vi "Valore da riga acq.vi"(10 "Filtro":bool[](array[boolean]), 11 "RIGA":string[](array[string])) -> (3 "MISURE NM":T1)   [LabVIEW 2019]
uses:
  TypeDef/MISURE NM.ctl
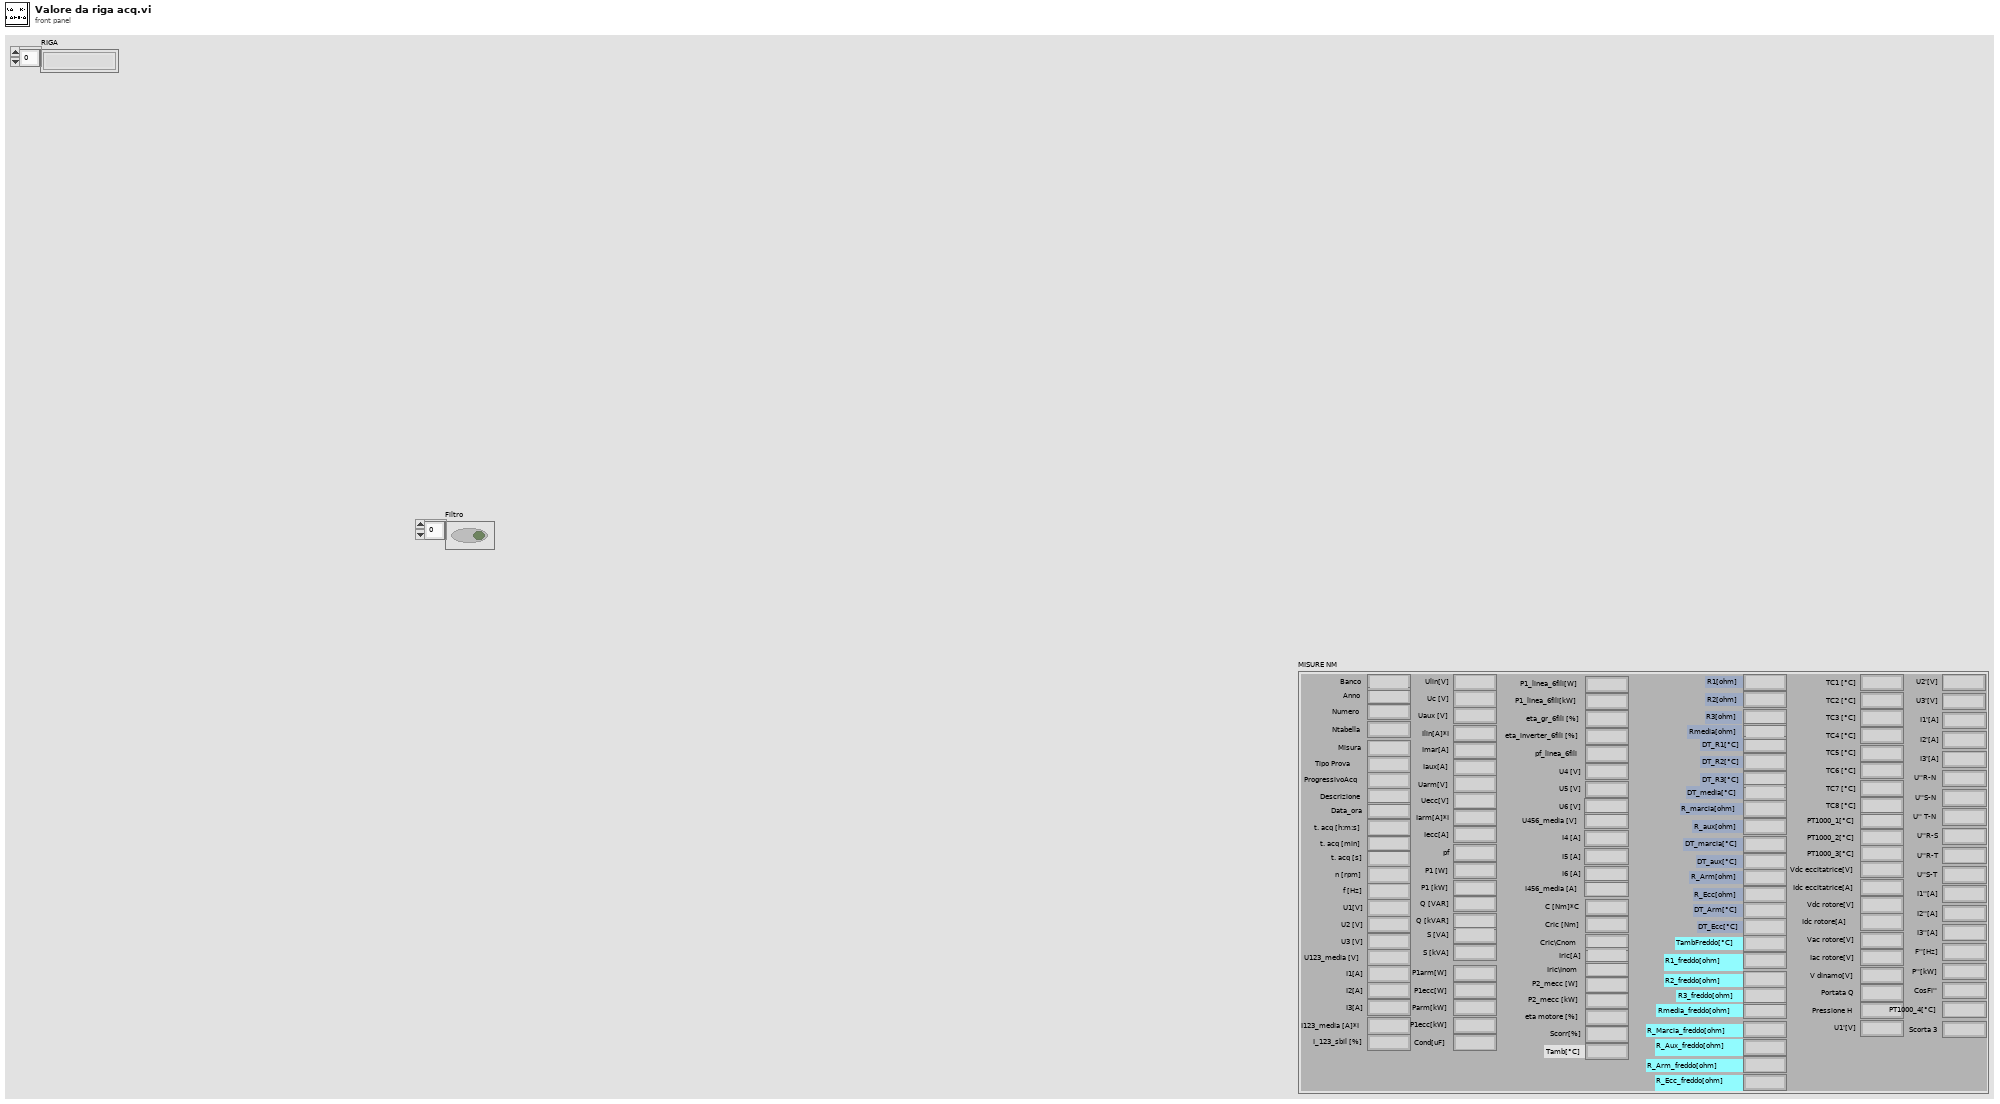
[diagram p1: front panel]
types:
  T1 = typedef "MISURE NM.ctl" = cluster{"Banco":string, "Anno":string, "Numero":string, "Ntabella":string, "Misura":string, "Tipo Prova":string, "ProgressivoAcq":string, "Descrizione":string, "Data_ora":string, "t. acq [h:m:s]":string, "t. acq [min]":string, "t. acq [s]":string, "n [rpm]":string, "f [Hz]":string, "U1[V]":string, "U2 [V]":string, "U3 [V]":string, "U123_media [V]":string, "I1[A]":string, "I2[A]":string, "I3[A]":string, "I123_media [A]*I":string, "I_123_sbil [%]":string, "Ulin[V]":string, "Uc [V]":string, "Uaux [V]":string, "Ilin[A]*I":string, "Imar[A]":string, "Iaux[A]":string, "Uarm[V]":string, "Uecc[V]":string, "Iarm[A]*I":string, "Iecc[A]":string, "pf":string, "P1 [W]":string, "P1 [kW]":string, "Q [VAR]":string, "Q [kVAR]":string, "S [VA]":string, "S [kVA]":string, "P1arm[W]":string, "P1ecc[W]":string, "Parm[kW]":string, "P1ecc[kW]":string, "Cond[uF]":string, "P1_linea_6fili[W]":string, "P1_linea_6fili[kW]":string, "eta_gr_6fili [%]":string, "eta_inverter_6fili [%]":string, "pf_linea_6fili":string, "U4 [V]":string, "U5 [V]":string, "U6 [V]":string, "U456_media [V]":string, "I4 [A]":string, "I5 [A]":string, "I6 [A]":string, "I456_media [A]":string, "C [Nm]*C":string, "Cric [Nm]":string, "Cric\\Cnom":string, "Iric[A]":string, "Iric\\Inom":string, "P2_mecc [W]":string, "P2_mecc [kW]":string, "eta motore [%]":string, "Scorr[%]":string, "Tamb[°C]":string, "R1[ohm]":string, "R2[ohm]":string, "R3[ohm]":string, "Rmedia[ohm]":string, "DT_R1[°C]":string, "DT_R2[°C]":string, "DT_R3[°C]":string, "DT_media[°C]":string, "R_marcia[ohm]":string, "R_aux[ohm]":string, "DT_marcia[°C]":string, "DT_aux[°C]":string, "R_Arm[ohm]":string, "R_Ecc[ohm]":string, "DT_Arm[°C]":string, "DT_Ecc[°C]":string, "TambFreddo[°C]":string, "R1_freddo[ohm]":string, "R2_freddo[ohm]":string, "R3_freddo[ohm]":string, "Rmedia_freddo[ohm]":string, "R_Marcia_freddo[ohm]":string, "R_Aux_freddo[ohm]":string, "R_Arm_freddo[ohm]":string, "R_Ecc_freddo[ohm]":string, "TC1 [°C]":string, "TC2 [°C]":string, "TC3 [°C]":string, "TC4 [°C]":string, "TC5 [°C]":string, "TC6 [°C]":string, "TC7 [°C]":string, "TC8 [°C]":string, "PT1000_1[°C]":string, "PT1000_2[°C]":string, "PT1000_3[°C]":string, "Vdc eccitatrice[V]":string, "Idc eccitatrice[A]":string, "Vdc rotore[V]":string, "Idc rotore[A]":string, "Vac rotore[V]":string, "Iac rotore[V]":string, "V dinamo[V]":string, "Portata Q":string, "Pressione H":string, "U1'[V]":string, "U2'[V]":string, "U3'[V]":string, "I1'[A]":string, "I2'[A]":string, "I3'[A]":string, "U''R-N":string, "U''S-N":string, "U'' T-N":string, "U''R-S":string, "U''R-T":string, "U''S-T":string, "I1''[A]":string, "I2''[A]":string, "I3''[A]":string, "F''[Hz]":string, "P''[kW]":string, "CosFi''":string, "PT1000_4[°C]":string, "Scorta 3":string}
  T2 = cluster{"[0]":string, "[1]":string, "[2]":string, "[3]":string, "[4]":string, "[5]":string, "[6]":string, "[7]":string, "[8]":string, "[9]":string, "[10]":string, "[11]":string, "[12]":string, "[13]":string, "[14]":string, "[15]":string, "[16]":string, "[17]":string, "[18]":string, "[19]":string, "[20]":string, "[21]":string, "[22]":string, "[23]":string, "[24]":string, "[25]":string, "[26]":string, "[27]":string, "[28]":string, "[29]":string, "[30]":string, "[31]":string, "[32]":string, "[33]":string, "[34]":string, "[35]":string, "[36]":string, "[37]":string, "[38]":string, "[39]":string, "[40]":string, "[41]":string, "[42]":string, "[43]":string, "[44]":string, "[45]":string, "[46]":string, "[47]":string, "[48]":string, "[49]":string, "[50]":string, "[51]":string, "[52]":string, "[53]":string, "[54]":string, "[55]":string, "[56]":string, "[57]":string, "[58]":string, "[59]":string, "[60]":string, "[61]":string, "[62]":string, "[63]":string, "[64]":string, "[65]":string, "[66]":string, "[67]":string, "[68]":string, "[69]":string, "[70]":string, "[71]":string, "[72]":string, "[73]":string, "[74]":string, "[75]":string, "[76]":string, "[77]":string, "[78]":string, "[79]":string, "[80]":string, "[81]":string, "[82]":string, "[83]":string, "[84]":string, "[85]":string, "[86]":string, "[87]":string, "[88]":string, "[89]":string, "[90]":string, "[91]":string, "[92]":string, "[93]":string, "[94]":string, "[95]":string, "[96]":string, "[97]":string, "[98]":string, "[99]":string, "[100]":string, "[101]":string, "[102]":string, "[103]":string, "[104]":string, "[105]":string, "[106]":string, "[107]":string, "[108]":string, "[109]":string, "[110]":string, "[111]":string, "[112]":string, "[113]":string, "[114]":string, "[115]":string, "[116]":string, "[117]":string, "[118]":string, "[119]":string, "[120]":string, "[121]":string, "[122]":string, "[123]":string, "[124]":string, "[125]":string, "[126]":string, "[127]":string, "[128]":string, "[129]":string, "[130]":string, "[131]":string, "[132]":string}
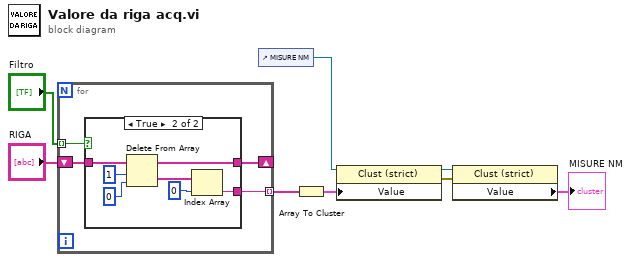
[diagram p0: block diagram]
diagram:
  n1 = for {
    shift-right: [w11] -> _
    shift-left: "RIGA" -> [w12]
    tunnel: "Filtro" -> [w10] mode=indexing
    tunnel: [w9] -> w7 mode=indexing
    n2 = case shown="True" w10 {
      tunnel: w12 -> [w13 w20]
      tunnel: [w13 w19] -> w11
      tunnel: [_ w17] -> w9
      frame False {
      }
      frame True {
        n3 = Delete From Array(array=w20, length=1, index=0 ("length")) -> (deleted portion=w18:string[], array with subset deleted=w19:string[])
        n4 = Index Array(array=w18, index=0 ("index (row)")) -> (element=w17:string)
      }
    }
  }
  n5 = control-ref of="MISURE NM"() -> (w1:refnum<vi>)
  n6 = Array To Cluster(array=w7) -> (cluster=w6:T2)
  n7 = property class="Clust (strict)"(reference=w1, "Value"=w6) -> (reference out=w5:refnum<vi>, error out=w4:errorcluster)  [unwired: 1 in]
  n8 = property class="Clust (strict)"(reference=w5, error in=w4) -> ("Value"=→"MISURE NM":T1)  [unwired: 2 out]
